vi "NI-Embedded CAN for RIO subVI - CAN Frame to Table2.vi"(5 "appended array":string[](array[string]), 6 "x":dbl, 7 "Hexadecimal?":bool, 8 "error in (no error)":errorcluster, 9 "timestamp":timestamp, 10 "CAN frame":T1 {"type" items=["CAN Data", "CAN Remote"]; "identifier" format="%.0x"}, 11 "Input Array":string[][](array[string])) -> (3 "Output Array":string[][](array[string]), 4 "Numeric":dbl)   [LabVIEW 2014]
doc: "This example shows how to put a CAN transceiver to sleep on RIO Embedded CAN devices."
uses:
  <vilib>/RioEmbeddedCAN/RioEmbeddedCAN.llb/CANFrameControl.ctl
panel:
  out "subarray 2":string[](array[string])
  out "subarray":string[](array[string])
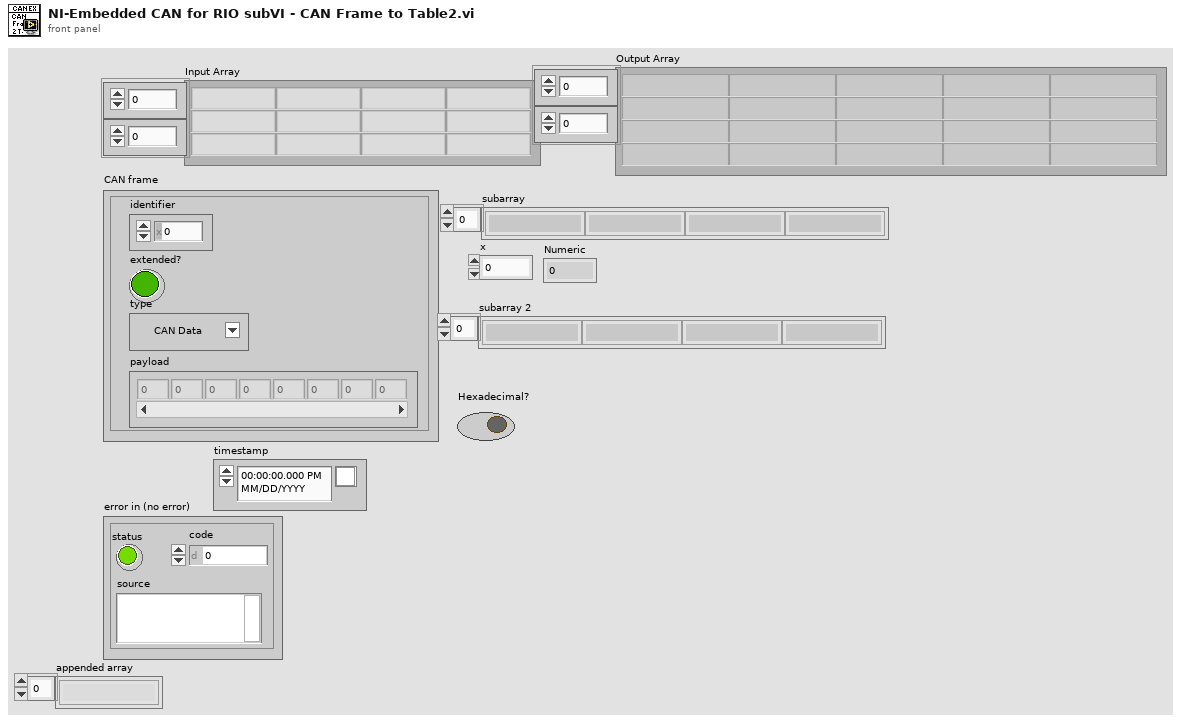
[diagram p1: front panel]
types:
  T1 = typedef "CANFrameControl.ctl" = cluster{"identifier":u32, "extended?":bool, "type":u8, "payload":u8[]}
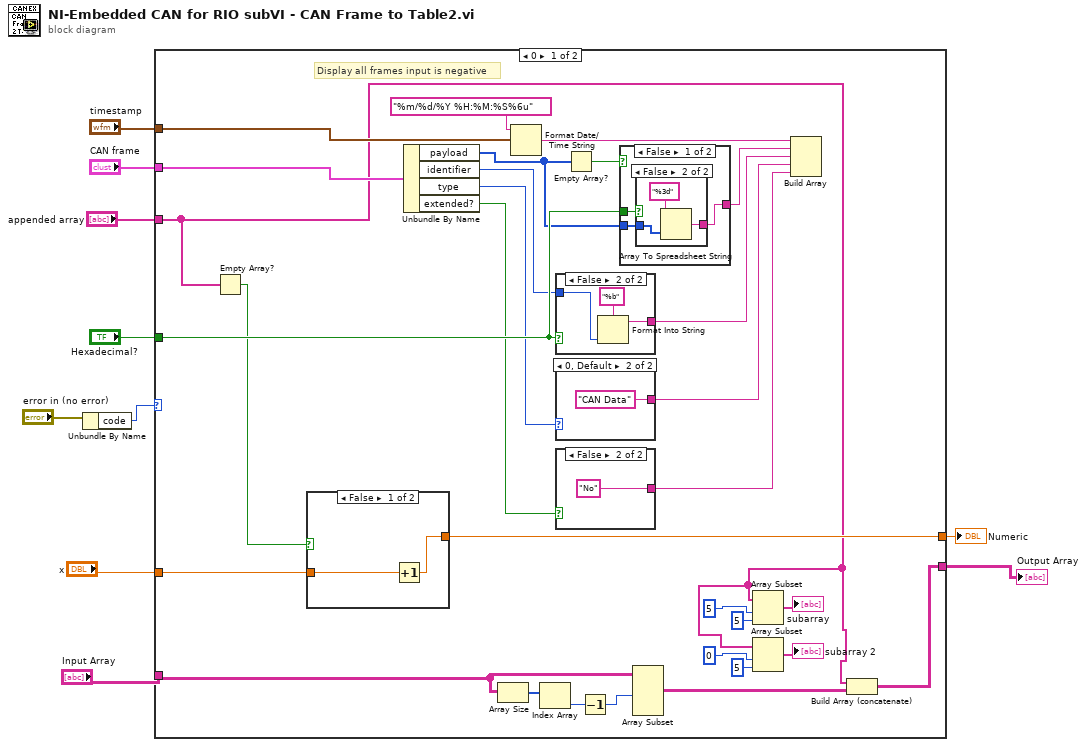
[diagram p0: block diagram]
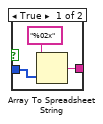
[diagram p3: hidden frame]
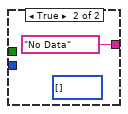
[diagram p4: hidden frame]
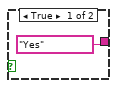
[diagram p5: hidden frame]
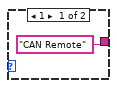
[diagram p6: hidden frame]
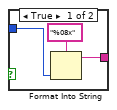
[diagram p7: hidden frame]
diagram:
  n1 = Unbundle By Name("error in (no error)") -> ("code"=w8:i32)
  n2 = case shown="0" w8 {
    tunnel: "Input Array" -> [w36 w65]
    tunnel: [w35 w65] -> w5
    tunnel: "Hexadecimal?" -> [w34 _]
    tunnel: "CAN frame" -> [w32 _]
    tunnel: "timestamp" -> [w33 _]
    tunnel: [w15 w64] -> w2
    tunnel: "x" -> [w14 w64]
    tunnel: "appended array" -> [w12 _]
    frame 0 {
      # "Display all frames input is negative"
      n3 = Empty Array?(array=w12) -> (empty?=w11:bool)
      n4 = case shown="False" w11 {
        tunnel: [w42 w43] -> w15
        tunnel: w14 -> [w41 w43]
        frame False {
          n5 = Increment(x=w41) -> (x+1=w42:dbl)
        }
        frame True {
        }
      }
      n6 = Unbundle By Name(w32) -> ("payload"=w17:u8[], "identifier"=w13:u32, "type"=w23:u8, "extended?"=w20:bool)
      n7 = Array Size(array=w36) -> (size(s)=w40:i32[])
      n8 = Format Date/Time String(time format string (%c)="%m/%d/%Y %H:%M:%S%6u", seconds (now)=w33) -> (date/time string=w25:string)  [unwired: 1 in]
      n9 = Index Array(array=w40) -> (element=w39:i32)  [unwired: 1 in]
      n10 = case shown="False" w34 {
        tunnel: w13 -> [w59 w62]
        tunnel: [w58 w61] -> w24
        frame True {
          n11 = Format Into String(format string="%08x", w59) -> (resulting string=w58:string)  [unwired: 2 in, 1 out]
        }
        frame False {
          n12 = Format Into String(format string="%b", w62) -> (resulting string=w61:string)  [unwired: 2 in, 1 out]
        }
      }
      n13 = case shown="0, Default" w23 {
        tunnel: ["CAN Remote" "CAN Data"] -> w22
        frame 1 {
        }
        frame 0, Default {
        }
      }
      n14 = case shown="False" w20 {
        tunnel: ["Yes" "No"] -> w21
        frame True {
        }
        frame False {
        }
      }
      n15 = Empty Array?(array=w17) -> (empty?=w16:bool)
      n16 = Decrement(x=w39) -> (x-1=w38:i32)
      n17 = case shown="False" w16 {
        tunnel: [w44 "No Data"] -> w19
        tunnel: w17 -> [w46 _]
        tunnel: w34 -> [w45 _]
        frame False {
          n18 = case shown="False" w45 {
            tunnel: w46 -> [w47 w50]
            tunnel: [w48 w51] -> w44
            frame True {
              n19 = Array To Spreadsheet String(array=w47, 3:"%02x" ("format string")) -> (spreadsheet string=w48:string)  [unwired: 1 in]
            }
            frame False {
              n20 = Array To Spreadsheet String(array=w50, 3:"%3d" ("format string")) -> (spreadsheet string=w51:string)  [unwired: 1 in]
            }
          }
        }
        frame True {
          (unwired) u8[] [] ("payload")
        }
      }
      n21 = Array Subset(array=w36, length (row)=w38) -> (w37:string[][])  [unwired: 3 in]
      n22 = Array Subset(array=w12, index=5 ("length"), length=5) -> (→"subarray":string[])
      n23 = Array Subset(array=w12, index=0 ("length"), length=5) -> (→"subarray 2":string[])
      n24 = Build Array(w25, w19, w24, w22, w21) -> ()  [unwired: 1 out]
      n25 = Build Array (concatenate)(w12, w37) -> (w35:string[][])
    }
    frame Default {
    }
  }
  "Output Array" <- w5
  "Numeric" <- w2
